vi "Workspace.UI.Update.Captions.vi"(7 "Diagnostic Protocol":T1, 8 "error in (no error)":errorcluster, 10 "Cmd":T3, 11 "UI.Refs":T2) -> (0 "error out":errorcluster)   [LabVIEW 2015, in "Diagnostics Addon Shared.lvlib"]
uses:
  Diagnostics Addon Shared.lvlib
  Types/Command.ctl
  Types/UI.Refs.ctl
  Types/Protocol.ctl
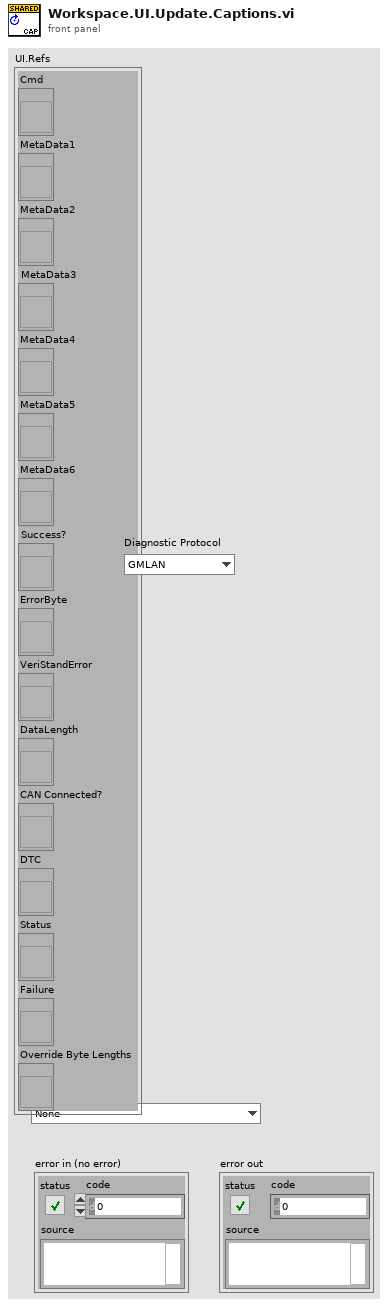
[diagram p1: front panel]
types:
  T1 = typedef "Diagnostics Addon Shared.lvlib/Protocol.ctl" = enum16{"GMLAN", "KWP-2000", "UDS", "User-Defined"}
  T2 = typedef "Diagnostics Addon Shared.lvlib/UI.Refs.ctl" = cluster{"Cmd":refnum<vi>, "MetaData1":refnum<vi>, "MetaData2":refnum<vi>, "MetaData3":refnum<vi>, "MetaData4":refnum<vi>, "MetaData5":refnum<vi>, "MetaData6":refnum<vi>, "Success?":refnum<vi>, "ErrorByte":refnum<vi>, "VeriStandError":refnum<vi>, "DataLength":refnum<vi>, "CAN Connected?":refnum<vi>, "DTC":refnum<vi>, "Status":refnum<vi>, "Failure":refnum<vi>, "Override Byte Lengths":refnum<vi>}
  T3 = typedef "Diagnostics Addon Shared.lvlib/Command.ctl" = enum8{"None", "EnableDiagnosticSession", "DisableDiagnosticSession", "ReadDataIdentifiers", "ReadDataIdentifier", "WriteDataIndentifier", "ReadPIDsOnDemand", "ReadPIDOnDemand", "WriteCPID", "WriteMemory", "ReadMemory", "ReadDTCs", "ClearDTCs", "ControlDTC", "ForceTesterPresent", "DisableNormalCommunication", "ReturnToNormalMode", "InputOutputControl", "StartRoutine", "RequestRoutineStatus", "StopRoutine", "ECUReset", "UnlockECU", "ClearSuccessBit", "ConfigureandStartPIDs", "StopPIDs", "StartDTCs", "EnableChangeDTCCount", "DisableChangeDTCCount", "ReadFailureRecordParameters", "PassThru Channel Based", "EnableRepeatingTesterPresent", "DisableRepeatingTesterPresent", "CloseCANCommunication", "RestartCANCommunication"}
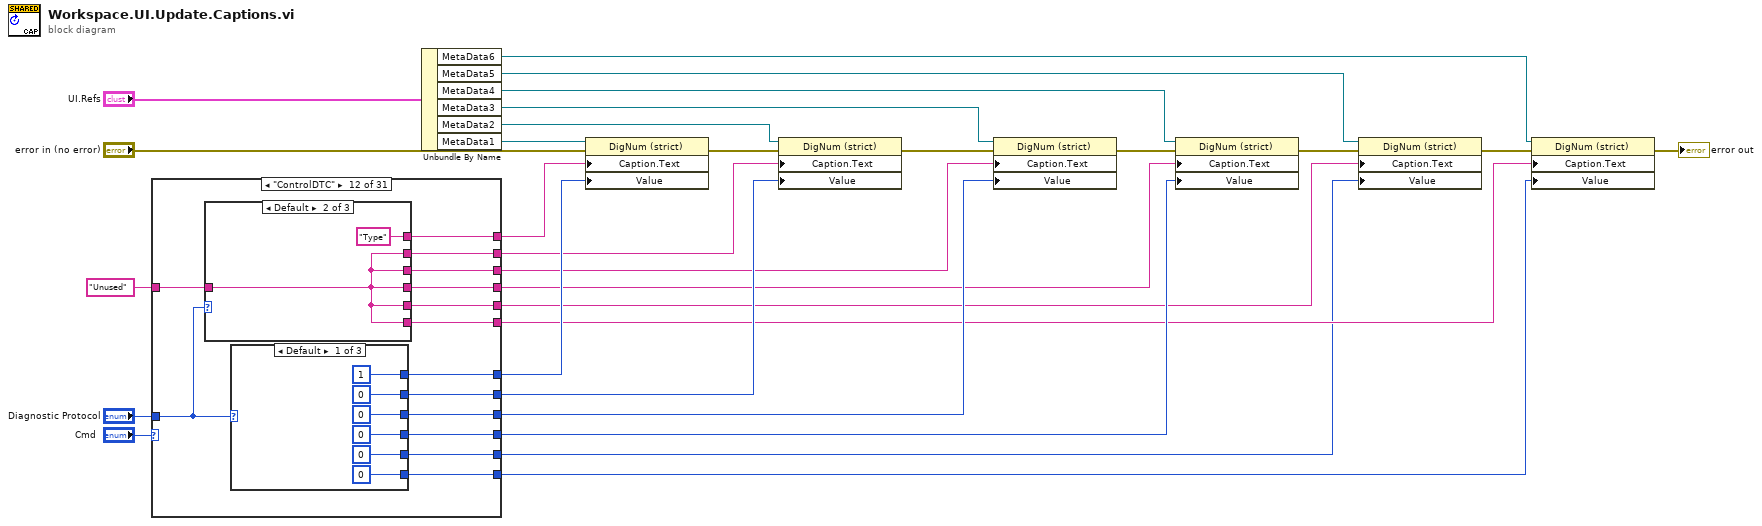
[diagram p0: block diagram]
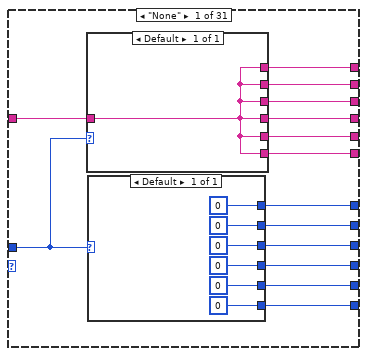
[diagram p2: hidden frame]
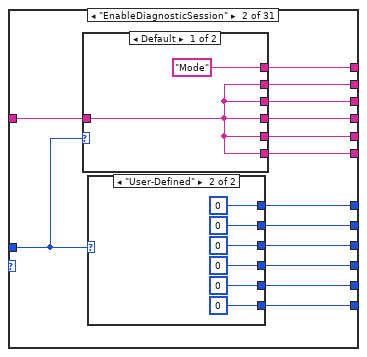
[diagram p3: hidden frame]
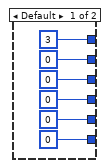
[diagram p5: hidden frame]
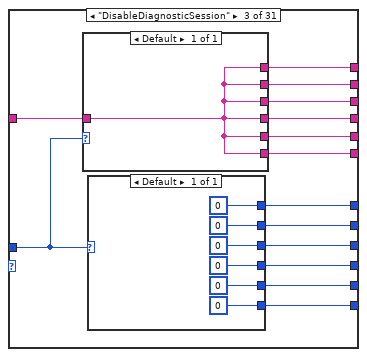
[diagram p6: hidden frame]
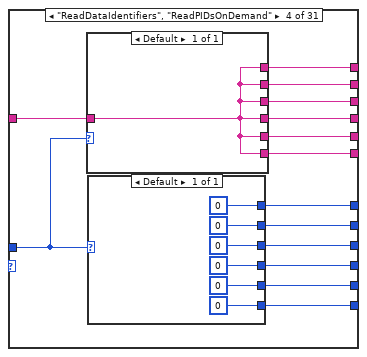
[diagram p7: hidden frame]
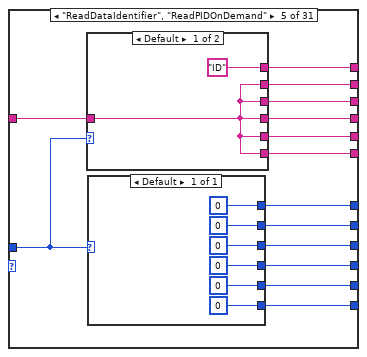
[diagram p8: hidden frame]
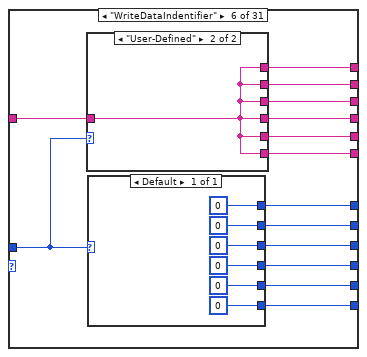
[diagram p10: hidden frame]
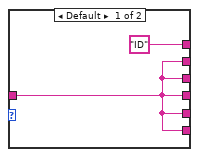
[diagram p11: hidden frame]
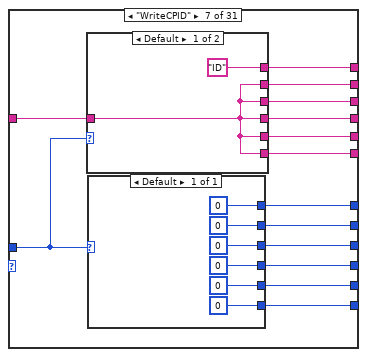
[diagram p12: hidden frame]
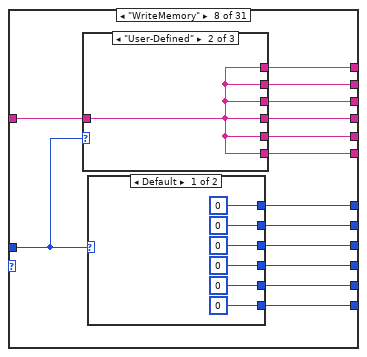
[diagram p14: hidden frame]
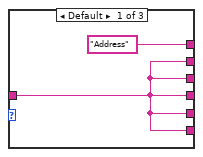
[diagram p15: hidden frame]
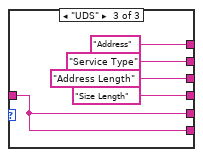
[diagram p16: hidden frame]
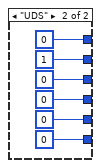
[diagram p17: hidden frame]
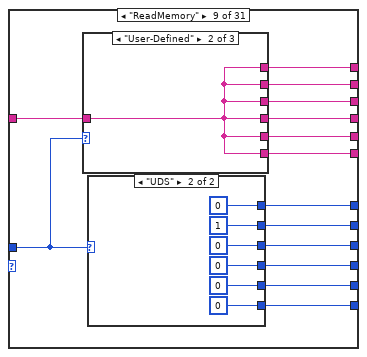
[diagram p18: hidden frame]
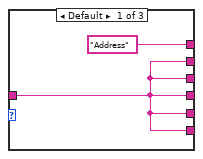
[diagram p19: hidden frame]
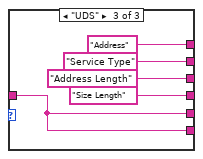
[diagram p20: hidden frame]
diagram:
  n1 = case shown="\"ControlDTC\"" "Cmd" {
    tunnel: [w39 w60 w89 w110 w131 w154 w177 w200 w234 w268 w316 w354 w394 w425 w457 w478 w514 w537 w566 w587 w608 w629 w650 w679 w701 w708 w722 w745 w770 w795 w816] -> w28
    tunnel: [w43 w64 w93 w114 w135 w158 w181 w204 w238 w272 w320 w358 w398 w429 w461 w482 w518 w541 w570 w591 w612 w633 w654 w683 i64 0 ("Value") i64 0 ("Value") w726 w749 w774 w799 w820] -> w29
    tunnel: [w37 w58 w87 w108 w129 w152 w175 w198 w232 w266 w314 w352 w392 w423 w455 w476 w512 w535 w564 w585 w606 w627 w648 w677 w701 w708 w720 w743 w768 w793 w814] -> w17
    tunnel: [w42 w63 w92 w113 w134 w157 w180 w203 w237 w271 w319 w357 w397 w428 w460 w481 w517 w540 w569 w590 w611 w632 w653 w682 i64 0 ("Value") i64 0 ("Value") w725 w748 w773 w798 w819] -> w16
    tunnel: [w35 w56 w85 w106 w127 w150 w173 w196 w230 w264 w312 w350 w390 w421 w453 w474 w510 w533 w562 w583 w604 w625 w646 w675 w701 w708 w718 w741 w766 w791 w812] -> w15
    tunnel: [w41 w62 w91 w112 w133 w156 w179 w202 w236 w270 w318 w356 w396 w427 w459 w480 w516 w539 w568 w589 w610 w631 w652 w681 i64 0 ("Value") i64 0 ("Value") w724 w747 w772 w797 w818] -> w14
    tunnel: [w34 w55 w84 w105 w126 w149 w172 w195 w229 w263 w311 w349 w389 w420 w452 w473 w509 w532 w561 w582 w603 w624 w645 w674 w701 w708 w717 w740 w765 w790 w811] -> w13
    tunnel: [w40 w61 w90 w111 w132 w155 w178 w201 w235 w269 w317 w355 w395 w426 w458 w479 w515 w538 w567 w588 w609 w630 w651 w680 i64 0 ("Value") i64 0 ("Value") w723 w746 w771 w796 w817] -> w12
    tunnel: "Unused" -> [w36 w57 w86 w107 w128 w151 w174 w197 w231 w265 w313 w351 w391 w422 w454 w475 w511 w534 w563 w584 w605 w626 w647 w676 w701 w708 w719 w742 w767 w792 w813]
    tunnel: "Diagnostic Protocol" -> [w38 w59 w88 w109 w130 w153 w176 w199 w233 w267 w315 w353 w393 w424 w456 w477 w513 w536 w565 w586 w607 w628 w649 w678 _ _ w721 w744 w769 w794 w815]
    tunnel: [w33 w52 w82 w101 w122 w147 w169 w193 w225 w260 w309 w347 w387 w418 w450 w471 w507 w530 w559 w580 w601 w622 w643 w672 w701 w708 w716 w739 w764 w789 w809] -> w4
    tunnel: [w32 w51 w83 w102 w123 w148 w168 w194 w226 w259 w310 w348 w388 w419 w451 w472 w508 w531 w560 w581 w602 w623 w644 w673 w701 w708 w715 w738 w763 w788 w810] -> w3
    tunnel: [w31 w54 w81 w104 w125 w146 w171 w192 w228 w262 w308 w346 w386 w417 w449 w470 w506 w529 w558 w578 w600 w621 w641 w671 i64 0 ("Value") i64 0 ("Value") w714 w737 w762 w787 w808] -> w2
    tunnel: [w30 w53 w80 w103 w124 w145 w170 w191 w227 w261 w307 w345 w385 w416 w448 w469 w505 w528 w557 w579 w599 w620 w642 w670 i64 0 ("Value") i64 0 ("Value") w713 w736 w761 w786 w807] -> w1
    frame "None" {
      n2 = case shown="Default" w38 {
        tunnel: [w44] -> w39
        tunnel: [w44] -> w37
        tunnel: w36 -> [w44]
        tunnel: [w44] -> w35
        tunnel: [w44] -> w34
        tunnel: [w44] -> w33
        tunnel: [w44] -> w32
        frame Default {
        }
      }
      n3 = case shown="Default" w38 {
        tunnel: [i64 0 ("Value")] -> w43
        tunnel: [i64 0 ("Value")] -> w42
        tunnel: [i64 0 ("Value")] -> w41
        tunnel: [i64 0 ("Value")] -> w40
        tunnel: [i64 0 ("Value")] -> w31
        tunnel: [i64 0 ("Value")] -> w30
        frame Default {
        }
      }
    }
    frame "EnableDiagnosticSession" {
      n4 = case shown="Default" w59 {
        tunnel: ["Mode" w67] -> w60
        tunnel: [w65 w67] -> w58
        tunnel: w57 -> [w65 w67]
        tunnel: [w65 w67] -> w56
        tunnel: [w65 w67] -> w55
        tunnel: [w65 w67] -> w52
        tunnel: [w65 w67] -> w51
        frame Default {
        }
        frame "User-Defined" {
        }
      }
      n5 = case shown="\"User-Defined\"" w59 {
        tunnel: [i64 3 ("Value") i64 0 ("Value")] -> w64
        tunnel: [i64 0 ("Value") i64 0 ("Value")] -> w63
        tunnel: [i64 0 ("Value") i64 0 ("Value")] -> w62
        tunnel: [i64 0 ("Value") i64 0 ("Value")] -> w61
        tunnel: [i64 0 ("Value") i64 0 ("Value")] -> w54
        tunnel: [i64 0 ("Value") i64 0 ("Value")] -> w53
        frame Default {
        }
        frame "User-Defined" {
        }
      }
    }
    frame "DisableDiagnosticSession" {
      n6 = case shown="Default" w88 {
        tunnel: [w94] -> w89
        tunnel: [w94] -> w87
        tunnel: w86 -> [w94]
        tunnel: [w94] -> w85
        tunnel: [w94] -> w84
        tunnel: [w94] -> w83
        tunnel: [w94] -> w82
        frame Default {
        }
      }
      n7 = case shown="Default" w88 {
        tunnel: [i64 0 ("Value")] -> w93
        tunnel: [i64 0 ("Value")] -> w92
        tunnel: [i64 0 ("Value")] -> w91
        tunnel: [i64 0 ("Value")] -> w90
        tunnel: [i64 0 ("Value")] -> w81
        tunnel: [i64 0 ("Value")] -> w80
        frame Default {
        }
      }
    }
    frame "ReadDataIdentifiers", "ReadPIDsOnDemand" {
      n8 = case shown="Default" w109 {
        tunnel: [w115] -> w110
        tunnel: [w115] -> w108
        tunnel: w107 -> [w115]
        tunnel: [w115] -> w106
        tunnel: [w115] -> w105
        tunnel: [w115] -> w102
        tunnel: [w115] -> w101
        frame Default {
        }
      }
      n9 = case shown="Default" w109 {
        tunnel: [i64 0 ("Value")] -> w114
        tunnel: [i64 0 ("Value")] -> w113
        tunnel: [i64 0 ("Value")] -> w112
        tunnel: [i64 0 ("Value")] -> w111
        tunnel: [i64 0 ("Value")] -> w104
        tunnel: [i64 0 ("Value")] -> w103
        frame Default {
        }
      }
    }
    frame "ReadDataIdentifier", "ReadPIDOnDemand" {
      n10 = case shown="Default" w130 {
        tunnel: ["ID" w138] -> w131
        tunnel: [w136 w138] -> w129
        tunnel: w128 -> [w136 w138]
        tunnel: [w136 w138] -> w127
        tunnel: [w136 w138] -> w126
        tunnel: [w136 w138] -> w123
        tunnel: [w136 w138] -> w122
        frame Default {
        }
        frame "User-Defined" {
        }
      }
      n11 = case shown="Default" w130 {
        tunnel: [i64 0 ("Value")] -> w135
        tunnel: [i64 0 ("Value")] -> w134
        tunnel: [i64 0 ("Value")] -> w133
        tunnel: [i64 0 ("Value")] -> w132
        tunnel: [i64 0 ("Value")] -> w125
        tunnel: [i64 0 ("Value")] -> w124
        frame Default {
        }
      }
    }
    frame "WriteDataIndentifier" {
      n12 = case shown="\"User-Defined\"" w153 {
        tunnel: ["ID" w161] -> w154
        tunnel: [w159 w161] -> w152
        tunnel: w151 -> [w159 w161]
        tunnel: [w159 w161] -> w150
        tunnel: [w159 w161] -> w149
        tunnel: [w159 w161] -> w148
        tunnel: [w159 w161] -> w147
        frame Default {
        }
        frame "User-Defined" {
        }
      }
      n13 = case shown="Default" w153 {
        tunnel: [i64 0 ("Value")] -> w158
        tunnel: [i64 0 ("Value")] -> w157
        tunnel: [i64 0 ("Value")] -> w156
        tunnel: [i64 0 ("Value")] -> w155
        tunnel: [i64 0 ("Value")] -> w146
        tunnel: [i64 0 ("Value")] -> w145
        frame Default {
        }
      }
    }
    frame "WriteCPID" {
      n14 = case shown="Default" w176 {
        tunnel: ["ID" w184] -> w177
        tunnel: [w182 w184] -> w175
        tunnel: w174 -> [w182 w184]
        tunnel: [w182 w184] -> w173
        tunnel: [w182 w184] -> w172
        tunnel: [w182 w184] -> w169
        tunnel: [w182 w184] -> w168
        frame Default {
        }
        frame "User-Defined" {
        }
      }
      n15 = case shown="Default" w176 {
        tunnel: [i64 0 ("Value")] -> w181
        tunnel: [i64 0 ("Value")] -> w180
        tunnel: [i64 0 ("Value")] -> w179
        tunnel: [i64 0 ("Value")] -> w178
        tunnel: [i64 0 ("Value")] -> w171
        tunnel: [i64 0 ("Value")] -> w170
        frame Default {
        }
      }
    }
    frame "WriteMemory" {
      n16 = case shown="\"User-Defined\"" w199 {
        tunnel: ["Address" w207 "Address"] -> w200
        tunnel: [w205 w207 "Service Type"] -> w198
        tunnel: w197 -> [w205 w207 w208]
        tunnel: [w205 w207 "Address Length"] -> w196
        tunnel: [w205 w207 "Size Length"] -> w195
        tunnel: [w205 w207 w208] -> w194
        tunnel: [w205 w207 w208] -> w193
        frame Default {
        }
        frame "User-Defined" {
        }
        frame "UDS" {
        }
      }
      n17 = case shown="Default" w199 {
        tunnel: [i64 0 ("Value") i64 0 ("Value")] -> w204
        tunnel: [i64 0 ("Value") i64 1 ("Value")] -> w203
        tunnel: [i64 0 ("Value") i64 0 ("Value")] -> w202
        tunnel: [i64 0 ("Value") i64 0 ("Value")] -> w201
        tunnel: [i64 0 ("Value") i64 0 ("Value")] -> w192
        tunnel: [i64 0 ("Value") i64 0 ("Value")] -> w191
        frame Default {
        }
        frame "UDS" {
        }
      }
    }
    frame "ReadMemory" {
      n18 = case shown="\"User-Defined\"" w233 {
        tunnel: ["Address" w241 "Address"] -> w234
        tunnel: [w239 w241 "Service Type"] -> w232
        tunnel: w231 -> [w239 w241 w242]
        tunnel: [w239 w241 "Address Length"] -> w230
        tunnel: [w239 w241 "Size Length"] -> w229
        tunnel: [w239 w241 w242] -> w226
        tunnel: [w239 w241 w242] -> w225
        frame Default {
        }
        frame "User-Defined" {
        }
        frame "UDS" {
        }
      }
      n19 = case shown="\"UDS\"" w233 {
        tunnel: [i64 0 ("Value") i64 0 ("Value")] -> w238
        tunnel: [i64 0 ("Value") i64 1 ("Value")] -> w237
        tunnel: [i64 0 ("Value") i64 0 ("Value")] -> w236
        tunnel: [i64 0 ("Value") i64 0 ("Value")] -> w235
        tunnel: [i64 0 ("Value") i64 0 ("Value")] -> w228
        tunnel: [i64 0 ("Value") i64 0 ("Value")] -> w227
        frame Default {
        }
        frame "UDS" {
        }
      }
    }
    frame "ReadDTCs" {
      n20 = case shown="\"UDS\"" w267 {
        tunnel: ["Extension" "DTC" w282 "Extension"] -> w268
        tunnel: ["Mask" "FailureTypeByte" w282 "Group of DTC"] -> w266
        tunnel: w265 -> [_ w279 w282 _]
        tunnel: ["Severity" w279 w282 "Mode"] -> w264
        tunnel: ["DTC Byte Length Override" w279 w282 "DTC Byte Length Override"] -> w263
        tunnel: ["Status Byte Length Override" w279 w282 "Status Byte Length Override"] -> w260
        tunnel: ["Failure Byte Length Override" w279 w282 "Failure Byte Length Override"] -> w259
        frame "UDS" {
        }
        frame "GMLAN" {
        }
        frame "User-Defined" {
        }
        frame "KWP-2000" {
        }
      }
      n21 = case shown="\"UDS\"" w267 {
        tunnel: [i64 2 ("Value") i64 0 ("Value") i64 24 ("Value")] -> w272
        tunnel: [i64 0 ("Value") i64 0 ("Value") i64 65280 ("Value")] -> w271
        tunnel: [i64 0 ("Value") i64 0 ("Value") i64 3 ("Value")] -> w270
        tunnel: [i64 0 ("Value") i64 0 ("Value") i64 0 ("Value")] -> w269
        tunnel: [i64 0 ("Value") i64 0 ("Value") i64 0 ("Value")] -> w262
        tunnel: [i64 0 ("Value") i64 0 ("Value") i64 0 ("Value")] -> w261
        frame "UDS" {
        }
        frame "GMLAN", "User-Defined" {
        }
        frame "KWP-2000" {
        }
      }
    }
    frame "ClearDTCs" {
      n22 = case shown="Default" w315 {
        tunnel: ["Group of DTC" w326] -> w316
        tunnel: ["DTC Byte Length Override" w326] -> w314
        tunnel: w313 -> [w324 w326]
        tunnel: ["Status Byte Length Override" w326] -> w312
        tunnel: ["Failure Byte Length Override" w326] -> w311
        tunnel: [w324 w326] -> w310
        tunnel: [w324 w326] -> w309
        frame Default {
        }
        frame "GMLAN", "User-Defined" {
        }
      }
      n23 = case shown="\"GMLAN\", \"User-Defined\"" w315 {
        tunnel: [i64 16777215 ("Value") i64 0 ("Value") i64 65280 ("Value")] -> w320
        tunnel: [i64 0 ("Value") i64 0 ("Value") i64 0 ("Value")] -> w319
        tunnel: [i64 0 ("Value") i64 0 ("Value") i64 0 ("Value")] -> w318
        tunnel: [i64 0 ("Value") i64 0 ("Value") i64 0 ("Value")] -> w317
        tunnel: [i64 0 ("Value") i64 0 ("Value") i64 0 ("Value")] -> w308
        tunnel: [i64 0 ("Value") i64 0 ("Value") i64 0 ("Value")] -> w307
        frame Default {
        }
        frame "GMLAN", "User-Defined" {
        }
        frame "KWP-2000" {
        }
      }
    }
    frame "ControlDTC" {
      n24 = case shown="Default" w353 {
        tunnel: ["Group of DTC" "Type" w366] -> w354
        tunnel: ["DTC Byte Length Override" w364 w366] -> w352
        tunnel: w351 -> [w362 w364 w366]
        tunnel: ["Status Byte Length Override" w364 w366] -> w350
        tunnel: ["Failure Byte Length Override" w364 w366] -> w349
        tunnel: [w362 w364 w366] -> w348
        tunnel: [w362 w364 w366] -> w347
        frame "KWP-2000" {
        }
        frame Default {
        }
        frame "GMLAN", "User-Defined" {
        }
      }
      n25 = case shown="Default" w353 {
        tunnel: [i64 1 ("Value") i64 0 ("Value") i64 65280 ("Value")] -> w358
        tunnel: [i64 0 ("Value") i64 0 ("Value") i64 0 ("Value")] -> w357
        tunnel: [i64 0 ("Value") i64 0 ("Value") i64 0 ("Value")] -> w356
        tunnel: [i64 0 ("Value") i64 0 ("Value") i64 0 ("Value")] -> w355
        tunnel: [i64 0 ("Value") i64 0 ("Value") i64 0 ("Value")] -> w346
        tunnel: [i64 0 ("Value") i64 0 ("Value") i64 0 ("Value")] -> w345
        frame Default {
        }
        frame "GMLAN", "User-Defined" {
        }
        frame "KWP-2000" {
        }
      }
    }
    frame "ForceTesterPresent" {
      n26 = case shown="\"GMLAN\"" w393 {
        tunnel: ["Require Response?" "TargetType" w403] -> w394
        tunnel: [w399 w401 w403] -> w392
        tunnel: w391 -> [w399 w401 w403]
        tunnel: [w399 w401 w403] -> w390
        tunnel: [w399 w401 w403] -> w389
        tunnel: [w399 w401 w403] -> w388
        tunnel: [w399 w401 w403] -> w387
        frame Default {
        }
        frame "GMLAN" {
        }
        frame "User-Defined" {
        }
      }
      n27 = case shown="Default" w393 {
        tunnel: [i64 1 ("Value") i64 0 ("Value")] -> w398
        tunnel: [i64 0 ("Value") i64 0 ("Value")] -> w397
        tunnel: [i64 0 ("Value") i64 0 ("Value")] -> w396
        tunnel: [i64 0 ("Value") i64 0 ("Value")] -> w395
        tunnel: [i64 0 ("Value") i64 0 ("Value")] -> w386
        tunnel: [i64 0 ("Value") i64 0 ("Value")] -> w385
        frame Default {
        }
        frame "User-Defined" {
        }
      }
    }
    frame "DisableNormalCommunication" {
      n28 = case shown="\"User-Defined\"" w424 {
        tunnel: ["Type" "TargetType" w435] -> w425
        tunnel: ["Comm Type" w433 w435] -> w423
        tunnel: w422 -> [w430 w433 w435]
        tunnel: [w430 w433 w435] -> w421
        tunnel: [w430 w433 w435] -> w420
        tunnel: [w430 w433 w435] -> w419
        tunnel: [w430 w433 w435] -> w418
        frame Default {
        }
        frame "GMLAN" {
        }
        frame "User-Defined" {
        }
      }
      n29 = case shown="Default" w424 {
        tunnel: [i64 1 ("Value") i64 0 ("Value")] -> w429
        tunnel: [i64 0 ("Value") i64 0 ("Value")] -> w428
        tunnel: [i64 0 ("Value") i64 0 ("Value")] -> w427
        tunnel: [i64 0 ("Value") i64 0 ("Value")] -> w426
        tunnel: [i64 0 ("Value") i64 0 ("Value")] -> w417
        tunnel: [i64 0 ("Value") i64 0 ("Value")] -> w416
        frame Default {
        }
        frame "User-Defined" {
        }
      }
    }
    frame "ReturnToNormalMode" {
      n30 = case shown="Default" w456 {
        tunnel: [w462] -> w457
        tunnel: [w462] -> w455
        tunnel: w454 -> [w462]
        tunnel: [w462] -> w453
        tunnel: [w462] -> w452
        tunnel: [w462] -> w451
        tunnel: [w462] -> w450
        frame Default {
        }
      }
      n31 = case shown="Default" w456 {
        tunnel: [i64 0 ("Value")] -> w461
        tunnel: [i64 0 ("Value")] -> w460
        tunnel: [i64 0 ("Value")] -> w459
        tunnel: [i64 0 ("Value")] -> w458
        tunnel: [i64 0 ("Value")] -> w449
        tunnel: [i64 0 ("Value")] -> w448
        frame Default {
        }
      }
    }
    frame "InputOutputControl" {
      n32 = case shown="Default" w477 {
        tunnel: ["ID" w486] -> w478
        tunnel: ["Mode" w486] -> w476
        tunnel: w475 -> [w483 w486]
        tunnel: [w483 w486] -> w474
        tunnel: [w483 w486] -> w473
        tunnel: [w483 w486] -> w472
        tunnel: [w483 w486] -> w471
        frame Default {
        }
        frame "User-Defined" {
        }
      }
      n33 = case shown="Default" w477 {
        tunnel: [i64 0 ("Value") i64 0 ("Value") i64 0 ("Value")] -> w482
        tunnel: [i64 3 ("Value") i64 0 ("Value") i64 7 ("Value")] -> w481
        tunnel: [i64 0 ("Value") i64 0 ("Value") i64 0 ("Value")] -> w480
        tunnel: [i64 0 ("Value") i64 0 ("Value") i64 0 ("Value")] -> w479
        tunnel: [i64 0 ("Value") i64 0 ("Value") i64 0 ("Value")] -> w470
        tunnel: [i64 0 ("Value") i64 0 ("Value") i64 0 ("Value")] -> w469
        frame Default {
        }
        frame "User-Defined" {
        }
        frame "KWP-2000" {
        }
      }
    }
    frame "StartRoutine".."StopRoutine" {
      n34 = case shown="\"User-Defined\"" w513 {
        tunnel: ["ID" w521] -> w514
        tunnel: [w519 w521] -> w512
        tunnel: w511 -> [w519 w521]
        tunnel: [w519 w521] -> w510
        tunnel: [w519 w521] -> w509
        tunnel: [w519 w521] -> w508
        tunnel: [w519 w521] -> w507
        frame Default {
        }
        frame "User-Defined" {
        }
      }
      n35 = case shown="Default" w513 {
        tunnel: [i64 0 ("Value")] -> w518
        tunnel: [i64 0 ("Value")] -> w517
        tunnel: [i64 0 ("Value")] -> w516
        tunnel: [i64 0 ("Value")] -> w515
        tunnel: [i64 0 ("Value")] -> w506
        tunnel: [i64 0 ("Value")] -> w505
        frame Default {
        }
      }
    }
    frame "ECUReset" {
      n36 = case shown="Default" w536 {
        tunnel: ["Mode" w544] -> w537
        tunnel: [w542 w544] -> w535
        tunnel: w534 -> [w542 w544]
        tunnel: [w542 w544] -> w533
        tunnel: [w542 w544] -> w532
        tunnel: [w542 w544] -> w531
        tunnel: [w542 w544] -> w530
        frame Default {
        }
        frame "User-Defined" {
        }
      }
      n37 = case shown="Default" w536 {
        tunnel: [i64 1 ("Value") i64 0 ("Value")] -> w541
        tunnel: [i64 0 ("Value") i64 0 ("Value")] -> w540
        tunnel: [i64 0 ("Value") i64 0 ("Value")] -> w539
        tunnel: [i64 0 ("Value") i64 0 ("Value")] -> w538
        tunnel: [i64 0 ("Value") i64 0 ("Value")] -> w529
        tunnel: [i64 0 ("Value") i64 0 ("Value")] -> w528
        frame Default {
        }
        frame "User-Defined" {
        }
      }
    }
    frame "UnlockECU" {
      n38 = case shown="Default" w565 {
        tunnel: [w571] -> w566
        tunnel: [w571] -> w564
        tunnel: w563 -> [w571]
        tunnel: [w571] -> w562
        tunnel: [w571] -> w561
        tunnel: [w571] -> w560
        tunnel: [w571] -> w559
        frame Default {
        }
      }
      n39 = case shown="Default" w565 {
        tunnel: [i64 0 ("Value")] -> w570
        tunnel: [i64 0 ("Value")] -> w569
        tunnel: [i64 0 ("Value")] -> w568
        tunnel: [i64 0 ("Value")] -> w567
        tunnel: [i64 0 ("Value")] -> w558
        tunnel: [i64 0 ("Value")] -> w557
        frame Default {
        }
      }
    }
    frame "ClearSuccessBit" {
      n40 = case shown="Default" w586 {
        tunnel: [w592] -> w587
        tunnel: [w592] -> w585
        tunnel: w584 -> [w592]
        tunnel: [w592] -> w583
        tunnel: [w592] -> w582
        tunnel: [w592] -> w581
        tunnel: [w592] -> w580
        frame Default {
        }
      }
      n41 = case shown="Default" w586 {
        tunnel: [i64 0 ("Value")] -> w591
        tunnel: [i64 0 ("Value")] -> w590
        tunnel: [i64 0 ("Value")] -> w589
        tunnel: [i64 0 ("Value")] -> w588
        tunnel: [i64 0 ("Value")] -> w578
        tunnel: [i64 0 ("Value")] -> w579
        frame Default {
        }
      }
    }
    frame "ConfigureandStartPIDs" {
      n42 = case shown="Default" w607 {
        tunnel: [w613] -> w608
        tunnel: [w613] -> w606
        tunnel: w605 -> [w613]
        tunnel: [w613] -> w604
        tunnel: [w613] -> w603
        tunnel: [w613] -> w602
        tunnel: [w613] -> w601
        frame Default {
        }
      }
      n43 = case shown="Default" w607 {
        tunnel: [i64 0 ("Value")] -> w612
        tunnel: [i64 0 ("Value")] -> w611
        tunnel: [i64 0 ("Value")] -> w610
        tunnel: [i64 0 ("Value")] -> w609
        tunnel: [i64 0 ("Value")] -> w600
        tunnel: [i64 0 ("Value")] -> w599
        frame Default {
        }
      }
    }
    frame "StopPIDs" {
      n44 = case shown="Default" w628 {
        tunnel: [w634] -> w629
        tunnel: [w634] -> w627
        tunnel: w626 -> [w634]
        tunnel: [w634] -> w625
        tunnel: [w634] -> w624
        tunnel: [w634] -> w623
        tunnel: [w634] -> w622
        frame Default {
        }
      }
      n45 = case shown="Default" w628 {
        tunnel: [i64 0 ("Value")] -> w633
        tunnel: [i64 0 ("Value")] -> w632
        tunnel: [i64 0 ("Value")] -> w631
        tunnel: [i64 0 ("Value")] -> w630
        tunnel: [i64 0 ("Value")] -> w621
        tunnel: [i64 0 ("Value")] -> w620
        frame Default {
        }
      }
    }
    frame "StartDTCs" {
      n46 = case shown="\"User-Defined\"" w649 {
        tunnel: ["Status Mask" w657] -> w650
        tunnel: [w655 w657] -> w648
        tunnel: w647 -> [w655 w657]
        tunnel: [w655 w657] -> w646
        tunnel: [w655 w657] -> w645
        tunnel: [w655 w657] -> w644
        tunnel: [w655 w657] -> w643
        frame Default {
        }
        frame "User-Defined" {
        }
      }
      n47 = case shown="Default" w649 {
        tunnel: [i64 2 ("Value") i64 0 ("Value")] -> w654
        tunnel: [i64 0 ("Value") i64 0 ("Value")] -> w653
        tunnel: [i64 0 ("Value") i64 0 ("Value")] -> w652
        tunnel: [i64 0 ("Value") i64 0 ("Value")] -> w651
        tunnel: [i64 0 ("Value") i64 0 ("Value")] -> w641
        tunnel: [i64 0 ("Value") i64 0 ("Value")] -> w642
        frame Default {
        }
        frame "User-Defined" {
        }
      }
    }
    frame "EnableChangeDTCCount" {
      n48 = case shown="\"User-Defined\"" w678 {
        tunnel: ["Status Mask" w686] -> w679
        tunnel: [w684 w686] -> w677
        tunnel: w676 -> [w684 w686]
        tunnel: [w684 w686] -> w675
        tunnel: [w684 w686] -> w674
        tunnel: [w684 w686] -> w673
        tunnel: [w684 w686] -> w672
        frame Default {
        }
        frame "User-Defined" {
        }
      }
      n49 = case shown="Default" w678 {
        tunnel: [i64 2 ("Value") i64 0 ("Value")] -> w683
        tunnel: [i64 0 ("Value") i64 0 ("Value")] -> w682
        tunnel: [i64 0 ("Value") i64 0 ("Value")] -> w681
        tunnel: [i64 0 ("Value") i64 0 ("Value")] -> w680
        tunnel: [i64 0 ("Value") i64 0 ("Value")] -> w671
        tunnel: [i64 0 ("Value") i64 0 ("Value")] -> w670
        frame Default {
        }
        frame "User-Defined" {
        }
      }
    }
    frame "CloseCANCommunication" {
    }
    frame "RestartCANCommunication" {
    }
    frame "DisableChangeDTCCount" {
      n50 = case shown="Default" w721 {
        tunnel: ["Status Mask" w729] -> w722
        tunnel: [w727 w729] -> w720
        tunnel: w719 -> [w727 w729]
        tunnel: [w727 w729] -> w718
        tunnel: [w727 w729] -> w717
        tunnel: [w727 w729] -> w716
        tunnel: [w727 w729] -> w715
        frame Default {
        }
        frame "User-Defined" {
        }
      }
      n51 = case shown="Default" w721 {
        tunnel: [i64 0 ("Value")] -> w726
        tunnel: [i64 0 ("Value")] -> w725
        tunnel: [i64 0 ("Value")] -> w724
        tunnel: [i64 0 ("Value")] -> w723
        tunnel: [i64 0 ("Value")] -> w714
        tunnel: [i64 0 ("Value")] -> w713
        frame Default {
        }
      }
    }
    frame "ReadFailureRecordParameters" {
      n52 = case shown="Default" w744 {
        tunnel: ["ID" w754] -> w745
        tunnel: ["Failure Type" w754] -> w743
        tunnel: w742 -> [w750 w754]
        tunnel: ["Failure Record Number" w754] -> w741
        tunnel: [w750 w754] -> w740
        tunnel: [w750 w754] -> w739
        tunnel: [w750 w754] -> w738
        frame Default {
        }
        frame "User-Defined" {
        }
      }
      n53 = case shown="Default" w744 {
        tunnel: [i64 0 ("Value")] -> w749
        tunnel: [i64 0 ("Value")] -> w748
        tunnel: [i64 0 ("Value")] -> w747
        tunnel: [i64 0 ("Value")] -> w746
        tunnel: [i64 0 ("Value")] -> w737
        tunnel: [i64 0 ("Value")] -> w736
        frame Default {
        }
      }
    }
    frame "PassThru Channel Based" {
      n54 = case shown="Default" w769 {
        tunnel: ["Service"] -> w770
        tunnel: ["Service Length"] -> w768
        tunnel: w767 -> [w775]
        tunnel: ["Data Length"] -> w766
        tunnel: ["Response Required"] -> w765
        tunnel: [w775] -> w764
        tunnel: [w775] -> w763
        frame Default {
        }
      }
      n55 = case shown="Default" w769 {
        tunnel: [i64 0 ("Value")] -> w774
        tunnel: [i64 1 ("Value")] -> w773
        tunnel: [i64 0 ("Value")] -> w772
        tunnel: [i64 1 ("Value")] -> w771
        tunnel: [i64 0 ("Value")] -> w762
        tunnel: [i64 0 ("Value")] -> w761
        frame Default {
        }
      }
    }
    frame "EnableRepeatingTesterPresent" {
      n56 = case shown="Default" w794 {
        tunnel: [w800] -> w795
        tunnel: [w800] -> w793
        tunnel: w792 -> [w800]
        tunnel: [w800] -> w791
        tunnel: [w800] -> w790
        tunnel: [w800] -> w789
        tunnel: [w800] -> w788
        frame Default {
        }
      }
      n57 = case shown="Default" w794 {
        tunnel: [i64 0 ("Value")] -> w799
        tunnel: [i64 0 ("Value")] -> w798
        tunnel: [i64 0 ("Value")] -> w797
        tunnel: [i64 0 ("Value")] -> w796
        tunnel: [i64 0 ("Value")] -> w787
        tunnel: [i64 0 ("Value")] -> w786
        frame Default {
        }
      }
    }
    frame "DisableRepeatingTesterPresent" {
      n58 = case shown="Default" w815 {
        tunnel: [w821] -> w816
        tunnel: [w821] -> w814
        tunnel: w813 -> [w821]
        tunnel: [w821] -> w812
        tunnel: [w821] -> w811
        tunnel: [w821] -> w810
        tunnel: [w821] -> w809
        frame Default {
        }
      }
      n59 = case shown="Default" w815 {
        tunnel: [i64 0 ("Value")] -> w820
        tunnel: [i64 0 ("Value")] -> w819
        tunnel: [i64 0 ("Value")] -> w818
        tunnel: [i64 0 ("Value")] -> w817
        tunnel: [i64 0 ("Value")] -> w808
        tunnel: [i64 0 ("Value")] -> w807
        frame Default {
        }
      }
    }
  }
  n60 = Unbundle By Name("UI.Refs") -> ("MetaData6"=w5:refnum<vi>, "MetaData5"=w6:refnum<vi>, "MetaData4"=w18:refnum<vi>, "MetaData3"=w19:refnum<vi>, "MetaData2"=w20:refnum<vi>, "MetaData1"=w26:refnum<vi>)
  n61 = property class="DigNum (strict)"(reference=w26, error in="error in (no error)", "Caption.Text"=w28, "Value"=w29) -> (error out=w23:errorcluster)  [unwired: 1 out]
  n62 = property class="DigNum (strict)"(reference=w20, error in=w23, "Caption.Text"=w17, "Value"=w16) -> (error out=w22:errorcluster)  [unwired: 1 out]
  n63 = property class="DigNum (strict)"(reference=w19, error in=w22, "Caption.Text"=w15, "Value"=w14) -> (error out=w21:errorcluster)  [unwired: 1 out]
  n64 = property class="DigNum (strict)"(reference=w18, error in=w21, "Caption.Text"=w13, "Value"=w12) -> (error out=w8:errorcluster)  [unwired: 1 out]
  n65 = property class="DigNum (strict)"(reference=w6, error in=w8, "Caption.Text"=w4, "Value"=w2) -> (error out=w9:errorcluster)  [unwired: 1 out]
  n66 = property class="DigNum (strict)"(reference=w5, error in=w9, "Caption.Text"=w3, "Value"=w1) -> (error out=→"error out":errorcluster)  [unwired: 1 out]
